vi "identification_subroutine.vi"(10 "OutputRate":u16, 11 "Ident Go":bool) -> (1 "n_periods":u16, 2 "order_prbs":i8, 3 "identdata":dbl[][](array[numeric]))   [LabVIEW 2016]
uses:
  <vilib>/FPGAPlugInAG/PXIe-7975R/niLvFpga_Open_PXIe-7975R.vi
  <vilib>/rvi/interface/common/dynamic/niFpgaDynamicAddResources.vi
  <vilib>/Utility/error.llb/Error Cluster From Error Code.vi
  <vilib>/rvi/errors/niLvFpgaAdjustHostInterfaceError.vi
  <vilib>/rvi/interface/common/niFpgaWaitOnOcc.vi
  <vilib>/FPGAPlugInAG/Dynamic/niLvFpga_Close_Dynamic.vi
  <vilib>/rvi/interface/nirviOpenFPGA/nirviOpenFPGA.xnode
  qnmController/FPGA Bitfiles/qnmController797_flexRio_qnmFPGA0417_rCN683wrzyE.lvbitx
  qnmController/qnmFPGA_0417.vi
  <vilib>/rvi/interface/nirviReadWriteControl/nirviReadWriteControl.xnode
  <vilib>/rvi/interface/nirviMethod/nirviMethod.xnode
  <vilib>/rvi/interface/nirviCloseFPGA/nirviCloseFPGA.xnode
  <vilib>/rvi/interface/Simulation/niFpgaSimulationCallBeginRW.vi
  <vilib>/FPGAPlugInAG/Dynamic/niLvFpga_ReadFifo_Dynamic.vi
  <vilib>/rvi/errors/niLvFpgaMergeErrorWithErrorCode.vi
  NiFpgaLv.dll
  <vilib>/FPGAPlugInAG/Dynamic/niLvFpga_ConfigureFifo_Dynamic.vi
panel:
  in  "idParams":T1={"prbsOrder"=13, "minimum"=0, "maximum"=32, "outputRate"=50000, "repetitions"=100}
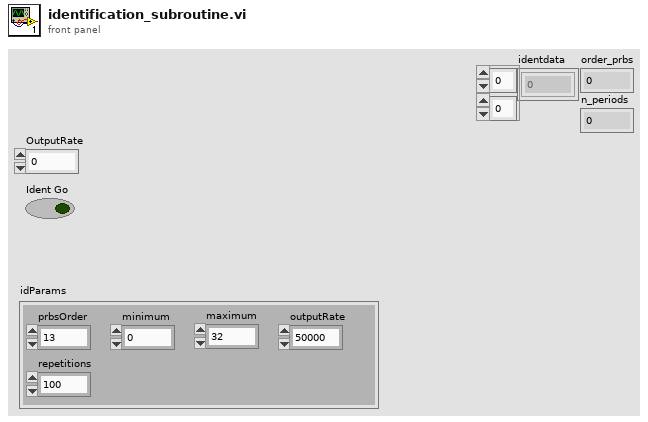
[diagram p1: front panel]
types:
  T1 = cluster{"prbsOrder":i8, "minimum":i16, "maximum":i16, "outputRate":u16, "repetitions":u16}
  T2 = cluster{"sysIdOutputRate":u16, "sysIdWaveSize":u16, "sysIdRepetitions":u16}
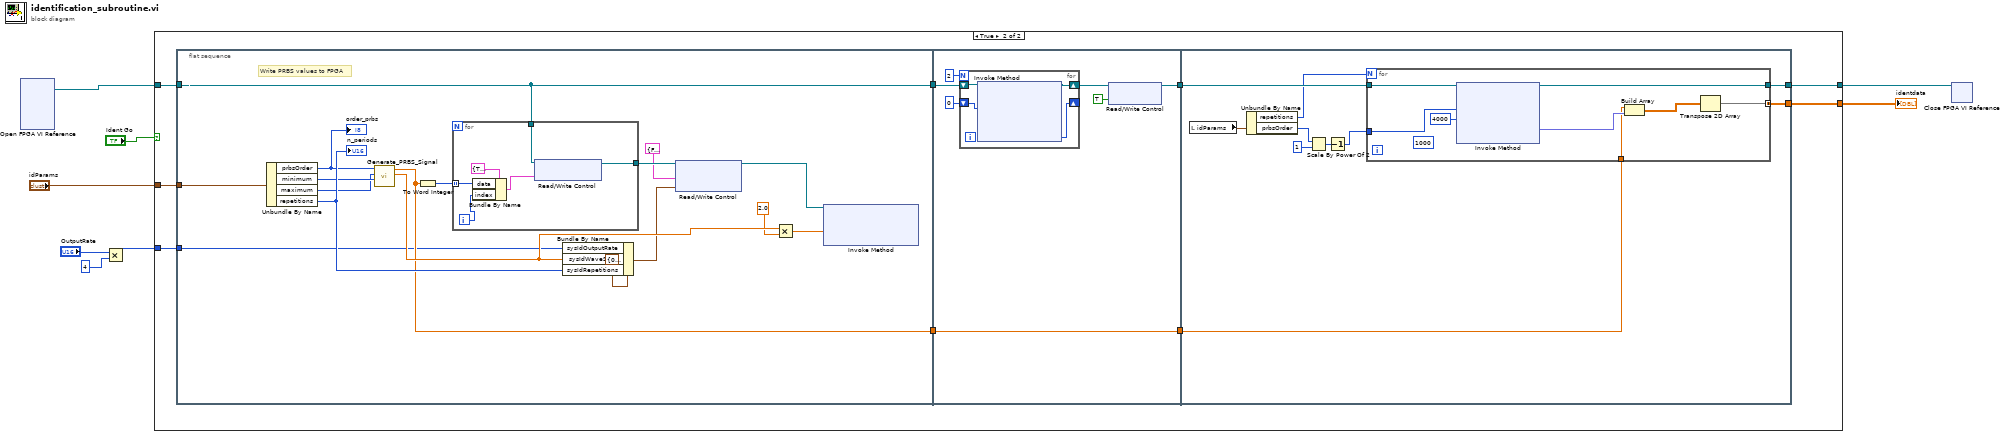
[diagram p0: block diagram]
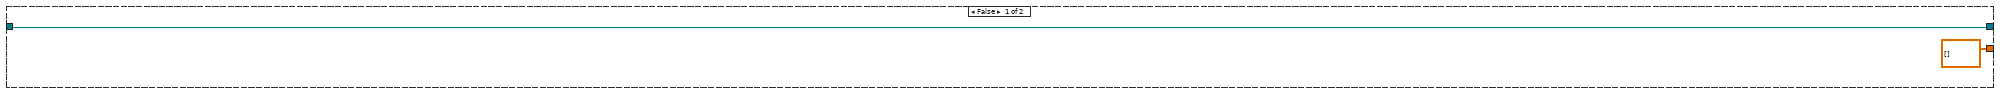
[diagram p2: hidden frame]
diagram:
  n1 = xnode "Open FPGA VI Reference"() -> ("FPGA VI Reference Out"=w8:refnum<k20>)  [unwired: 2 in, 1 out]
  n2 = Multiply(x="OutputRate", y=u16 4) -> (x*y=w5:u16)
  n3 = case shown="True" "Ident Go" {
    tunnel: w8 -> [w9 w18]
    tunnel: w5 -> [_ w14]
    tunnel: "idParams" -> [_ w13]
    tunnel: [dbl[][] [] w12] -> w2
    tunnel: [w9 w11] -> w1
    frame False {
    }
    frame True {
      n4 = flat-sequence {
        tunnel: w18 -> [w21]
        tunnel: [w21] -> w17
        tunnel: [w23] -> w16
        tunnel: w14 -> [w22]
        tunnel: w13 -> [w20]
        tunnel: [w47] -> w19
        tunnel: w17 -> [w49]
        tunnel: w16 -> [w43]
        tunnel: [w43] -> w15
        tunnel: w19 -> [w63]
        tunnel: [w56] -> w12
        tunnel: w15 -> [w55]
        tunnel: [w54] -> w11
        frame #0 {
          # "Write PRBS values to FPGA"
          n5 = Unbundle By Name(w20) -> ("prbsOrder"=w24:i8, "minimum"=w26:i16, "maximum"=w25:i16, "repetitions"=w34:u16)
          "order_prbs" <- w24
          "n_periods" <- w34
          n6 = call "Generate_PRBS_Signal.vi"("Min.Value"=w26, "Max. Value"=w25, "PRBS Order"=w24) -> ("PRBS Signal Length"=w36:dbl, "PRBS Signal"=w23:dbl[])  [unwired: 7 in]
          n7 = To Word Integer(number=w23) -> (16bit integer=w29:i16[])
          n8 = for {
            tunnel: w29 -> [w39] mode=indexing
            tunnel: [w38] -> w28
            tunnel: w21 -> [w37]
            i -> [w40]
            n9 = Bundle By Name(cluster=cluster{"write":bool, "data":i16, "index":u16} {"write"=TRUE, "data"=0, "index"=0} ("input cluster"), "data"=w39, "index"=w40) -> (w41:cluster{"write":bool, "data":i16, "index":u16})
            n10 = xnode "Read/Write Control"("FPGA VI Reference In"=w37, "sysIdWaveWrite"=w41) -> ("FPGA VI Reference Out"=w38:refnum<k20>)  [unwired: 1 in, 1 out]
          }
          n11 = Bundle By Name(cluster=T2 {"sysIdOutputRate"=0, "sysIdWaveSize"=0, "sysIdRepetitions"=0} ("sysIdParams"), "sysIdOutputRate"=w22, "sysIdWaveSize"=w36, "sysIdRepetitions"=w34) -> (w35:T2)
          n12 = xnode "Read/Write Control"("FPGA VI Reference In"=w28, "sysIdWaveWrite"=cluster{"write":bool, "data":i16, "index":u16} {"write"=FALSE, "data"=0, "index"=0} ("input cluster"), "sysIdParams"=w35) -> ("FPGA VI Reference Out"=w30:refnum<k20>)  [unwired: 1 in, 1 out]
          n13 = Multiply(x=w36, y=2.0) -> (x*y=w31:dbl)
          n14 = xnode "Invoke Method"("FPGA VI Reference In"=w30, "Requested Depth"=w31) -> ()  [unwired: 1 in, 3 out]
        }
        frame #1 {
          n15 = for {
            N: 2 -> [_]
            shift-right: [w52] -> w46
            shift-left: w49 -> [w53]
            shift-right: [w51] -> _
            shift-left: u32 0 ("Elements Remaining") -> [w50]
            n16 = xnode "Invoke Method"("FPGA VI Reference In"=w53, "Number of Elements"=w50) -> ("FPGA VI Reference Out"=w52:refnum<k20>, "Elements Remaining"=w51:u32)  [unwired: 2 in, 2 out]
          }
          n17 = xnode "Read/Write Control"("FPGA VI Reference In"=w46, "doSystemId"=TRUE) -> ("FPGA VI Reference Out"=w47:refnum<k20>)  [unwired: 1 in, 1 out]
        }
        frame #2 {
          n18 = local read "idParams"() -> (w62:T1)
          n19 = Unbundle By Name(w62) -> ("repetitions"=w57:u16, "prbsOrder"=w61:i8)
          n20 = Scale By Power Of 2(n=w61, x=i16 1) -> (x*2^n=w59:i16)
          n21 = Decrement(x=w59) -> (x-1=w58:i16)
          n22 = for {
            N: w57 -> [_]
            tunnel: w63 -> [w71]
            tunnel: w58 -> [w70]
            tunnel: [w64] -> w56 mode=concatenating
            tunnel: w55 -> [w67]
            tunnel: [w65] -> w54
            (unwired) 1000 ("Timeout (ms)")
            n23 = xnode "Invoke Method"("FPGA VI Reference In"=w71, "Number of Elements"=w70, "Timeout (ms)"=4000) -> ("FPGA VI Reference Out"=w65:refnum<k20>, "Data"=w68:fxp<+/-,24,16>[])  [unwired: 1 in, 2 out]
            n24 = Build Array(w67, w68) -> (w66:dbl[][])
            n25 = Transpose 2D Array(2D array=w66) -> (transposed array=w64:dbl[][])
          }
        }
      }
    }
  }
  "identdata" <- w2
  n26 = xnode "Close FPGA VI Reference"("FPGA VI Reference In"=w1) -> ()  [unwired: 1 in, 1 out]
